vi "Match Multiple Patterns.vi"(0 "string":string, 1 "upper limit (Inf)":i32=2147483647, 2 "regular expression":string[](array[string]), 3 "offset (0)":i32, 4 "lower limit (0)":i32) -> (6 "before substring":string, 7 "match substring":string, 8 "regular expression index":i32, 9 "after substring":string, 10 "offset past match":i32)   [LabVIEW 2021, in "Strings.lvlib"]
uses:
  Strings.lvlib
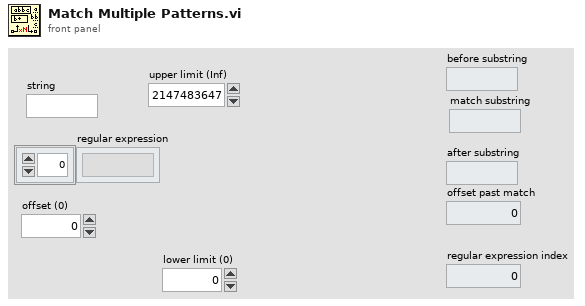
[diagram p1: front panel]
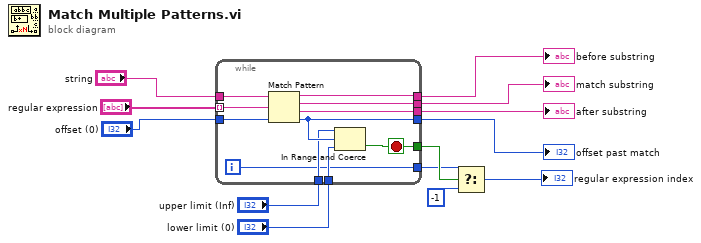
[diagram p0: block diagram]
diagram:
  n1 = while {
    tunnel: [w24] -> w12
    tunnel: [w23] -> w11
    tunnel: "regular expression" -> [w19] mode=indexing
    tunnel: "offset (0)" -> [w20]
    tunnel: [w18] -> w13
    tunnel: "string" -> [w22]
    tunnel: [w21] -> w9
    tunnel: "lower limit (0)" -> [w17]
    tunnel: "upper limit (Inf)" -> [w16]
    tunnel: [w15] -> w3
    tunnel: [w14] -> w4
    i -> [w15]
    stop <- w14 stop-if-true
    n2 = Match Pattern(string=w22, regular expression=w19, offset (0)=w20) -> (before substring=w21:string, match substring=w23:string, after substring=w24:string, offset past match=w18:i32)
    n3 = In Range and Coerce(upper limit=w16, x=w18, lower limit=w17) -> (In Range?=w14:bool)  [unwired: 1 out]
  }
  "before substring" <- w9
  "match substring" <- w11
  "after substring" <- w12
  "offset past match" <- w13
  n4 = Select(t=w3, s=w4, f=-1) -> (s? t:f=→"regular expression index":i32)
